vi "dipole_voltage_control_logic(SubVI).vi"(0 "CH1 Voltage":dbl=3.0, 1 "CH2 Voltage":dbl=5.0, 2 "positive":bool, 3 "off":bool, 4 "negative":bool) -> ()   [LabVIEW 2016]
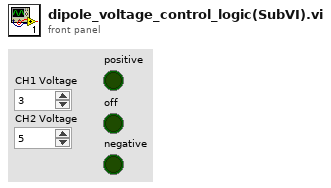
[diagram p1: front panel]
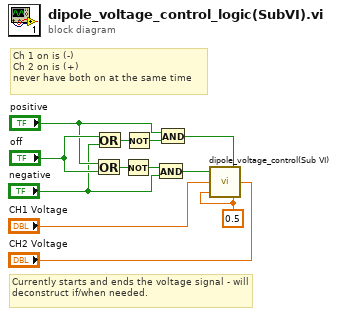
[diagram p0: block diagram]
diagram:
  w12 = 0.5 ("CH2 Current")
  # "Currently starts and ends the voltage signal - will deconstruct if/when needed."
  # "Ch 1 on is (-)\nCh 2 on is (+)\nnever have both on at the same time"
  n1 = Or(x="positive", y="off") -> (x .or. y?=w8:bool)
  n2 = Or(x="off", y="negative") -> (x .or. y?=w11:bool)
  n3 = Not(x=w8) -> (.not. x?=w4:bool)
  n4 = Not(x=w11) -> (.not. x?=w10:bool)
  n5 = And(x=w4, y="negative") -> (x .and. y?=w3:bool)
  n6 = And(x="positive", y=w10) -> (x .and. y?=w9:bool)
  n7 = call "dipole_voltage_control(Sub VI).vi"("CH2 Current"=w12, "CH2 Voltage"="CH2 Voltage", "CH2 enabled"=w9, "CH1 Current"=w12, "CH1 Voltage"="CH1 Voltage", "CH1 enabled"=w3) -> ()
